vi "write_local_status.vi"(8 "Argument":u8, 11 "Status code":T1) -> ()   [LabVIEW 2012]
uses:
  Common/i2c_status.ctl
  <vilib>/rvi/DataTransferAndStorage/Container/Common/niFpgaContainerExecOnDevCompGetState.vi
  <vilib>/rvi/Emulation/niFpgaSctlEmulationGetInTimedLoop.vi
  <vilib>/rvi/DataTransferAndStorage/Container/Common/niFpgaContainerGetUniqueNameForEmu.vi
  <vilib>/rvi/FIFO/Fifo_Resource/nirvififoEmulationSetSize.vi
  <vilib>/rvi/errors/niFpgaSetErrorForExecOnDevCompSimple.vi
  <vilib>/rvi/eio/common/nirviEmuReportErrorAndStop.vi
  <vilib>/rvi/Emulation/niFpgaSctlEmulationFifoFullMgr.vi
  <vilib>/rvi/Emulation/niFpgaSctlEmulationResourceMgr.vi
  <vilib>/rvi/interface/RandomDataEmulation/nirviRandomDataFPGAFIFO.vi
  <vilib>/rvi/interface/RandomDataEmulation/niFpgaRandomDataHandleErrors.vi
  <vilib>/rvi/DataTransferAndStorage/Container/XNode/niFpgaContainer.xnode
  <vilib>/rvi/FIFO/Fifo_Resource/niFpgaFifoEmulationRefIn.vi
panel:
  # "Number of bytes (1..255)"
  # "Stuff a status packet into the local read FIFO (pseudo-bus 3)"
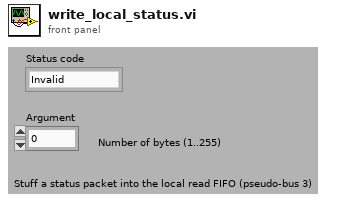
[diagram p1: front panel]
types:
  T1 = typedef "i2c_status.ctl" = enum8{"Invalid", "Command", "I2C start", "Trigger wait", "TX data wait", "Sequence", "Receive data", "I2C error", "Address NACK", "Data NACK", "SDA stuck", "SCL stuck", "Bad command"}
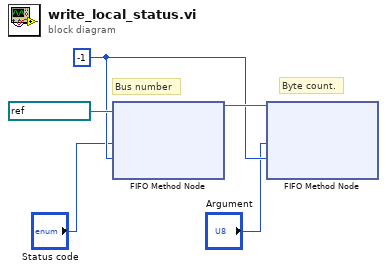
[diagram p0: block diagram]
diagram:
  w3 = -1 ("Timeout")
  # "Byte count."
  # "Bus number"
  n1 = xnode ("FIFO Method Node")("Element"="Status code", "Timeout"=w3, "FIFO In"=refnum<k21> "Local read" ("FIFO")) -> ("FIFO Out"=w4:refnum<k21>)  [unwired: 1 out]
  n2 = xnode ("FIFO Method Node")("Element"="Argument", "Timeout"=w3, "FIFO In"=w4) -> ()  [unwired: 2 out]
